vi "Commit Multiple Hardware Relay States.vi"(0 "RelayInterface in":refnum<class "RelayInterface.lvclass">, 5 "session in":refnum<k21>, 7 "device in":refnum<k21>, 9 "Commit String":string, 11 "error in (no error)":errorcluster) -> (4 "RelayInterface out":refnum<class "RelayInterface.lvclass">, 6 "session out":refnum<k21>, 8 "device out":refnum<k21>, 15 "error out":errorcluster)   [LabVIEW 2015, in "RelayInterface.lvclass"]
uses:
  RelayInterface.lvclass
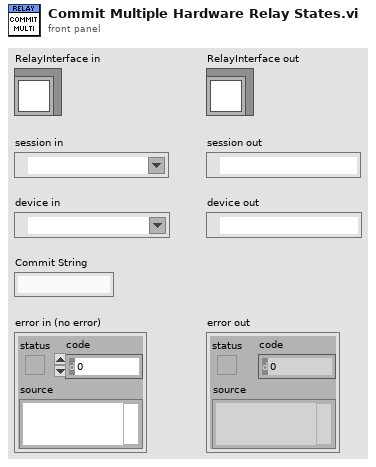
[diagram p1: front panel]
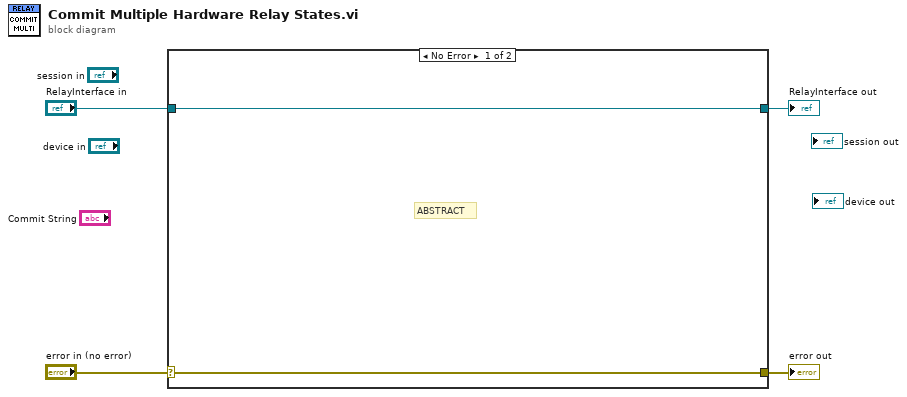
[diagram p0: block diagram]
diagram:
  n1 = case shown="No Error" "error in (no error)" {
    selector: "error in (no error)" -> [w6 w8]
    tunnel: [w6 w8] -> w3
    tunnel: [w5 w7] -> w1
    tunnel: "RelayInterface in" -> [w5 w7]
    frame No Error {
      # "ABSTRACT"
    }
    frame Error {
    }
  }
  "error out" <- w3
  "RelayInterface out" <- w1
